vi "test-translation3d.vi"(8 "error in (no error)":errorcluster) -> (0 "error out":errorcluster, 3 "All PASSED":bool)   [LabVIEW 2019]
uses:
  <vilib>/Rock Robotics/WPI/ThirdParty/JAS_Junk/TrajLib/VI/Quaternion_New.vi
  <vilib>/Rock Robotics/WPI/ThirdParty/JAS_Junk/TrajLib/VI/Rotation3d_Create_Default.vi
  <vilib>/Rock Robotics/WPI/ThirdParty/JAS_Junk/TrajLib/VI/Vector_Norm.vi
  <vilib>/Rock Robotics/WPI/ThirdParty/JAS_Junk/TrajLib/VecBuilder_ArrayBy1Fill.vi
  <vilib>/Rock Robotics/WPI/ThirdParty/JAS_Junk/TrajLib/VI/Rotation3d_GetQuaterion.vi
  <vilib>/Rock Robotics/WPI/ThirdParty/JAS_Junk/TrajLib/VI/Quaternion_Times.vi
  <vilib>/Rock Robotics/WPI/ThirdParty/JAS_Junk/TrajLib/VI/Quaternion_Inverse.vi
  <vilib>/Rock Robotics/WPI/ThirdParty/JAS_Junk/TrajLib/VI/Quaternion_Get_All.vi
  <vilib>/Rock Robotics/WPI/ThirdParty/JAS_Junk/TrajLib/VI/Quaternion_New_Default.vi
  <vilib>/Rock Robotics/WPI/ThirdParty/JAS_Junk/TrajLib/MatBuilder_Create.vi
  <vilib>/Rock Robotics/WPI/ThirdParty/JAS_Junk/TrajLib/Trajectory_Library.lvlib
panel:
  out "Test 7 Nearest To":bool
  out "Test 6":bool
  out "Test 3c":bool
  out "Test 3b":bool
  out "Test 3a":bool
  # "Translation3d"
  # "Didn't implement divide"
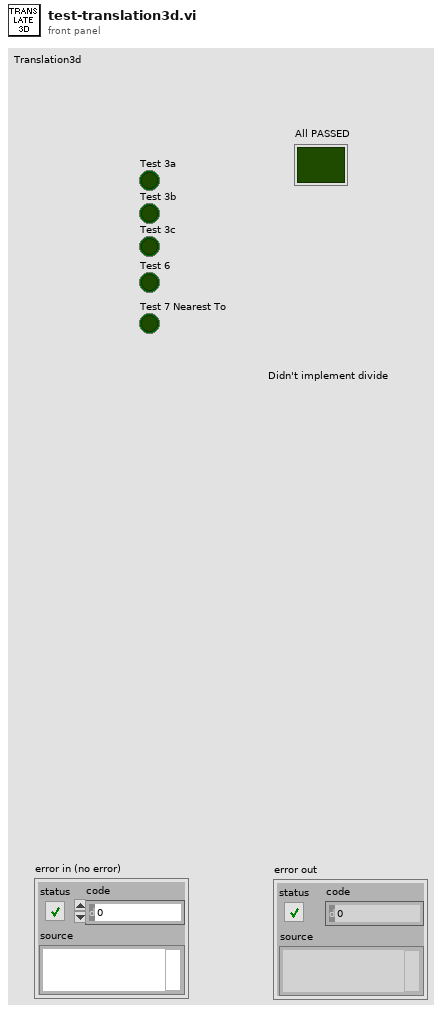
[diagram p1: front panel]
types:
  T1 = typedef "Trajectory_Library.lvlib/TRANSLATION3D.ctl" = cluster{"X":dbl, "Y":dbl, "Z":dbl}
  T2 = typedef "Trajectory_Library.lvlib/ROTATION3D.ctl" = cluster{"Q_quaternion":T3}
  T3 = typedef "Trajectory_Library.lvlib/QUATERNION.ctl" = cluster{"R":dbl, "V":dbl[]}
  T4 = typedef "Trajectory_Library.lvlib/TRANSLATION2D.ctl" = cluster{"X":dbl, "Y":dbl}
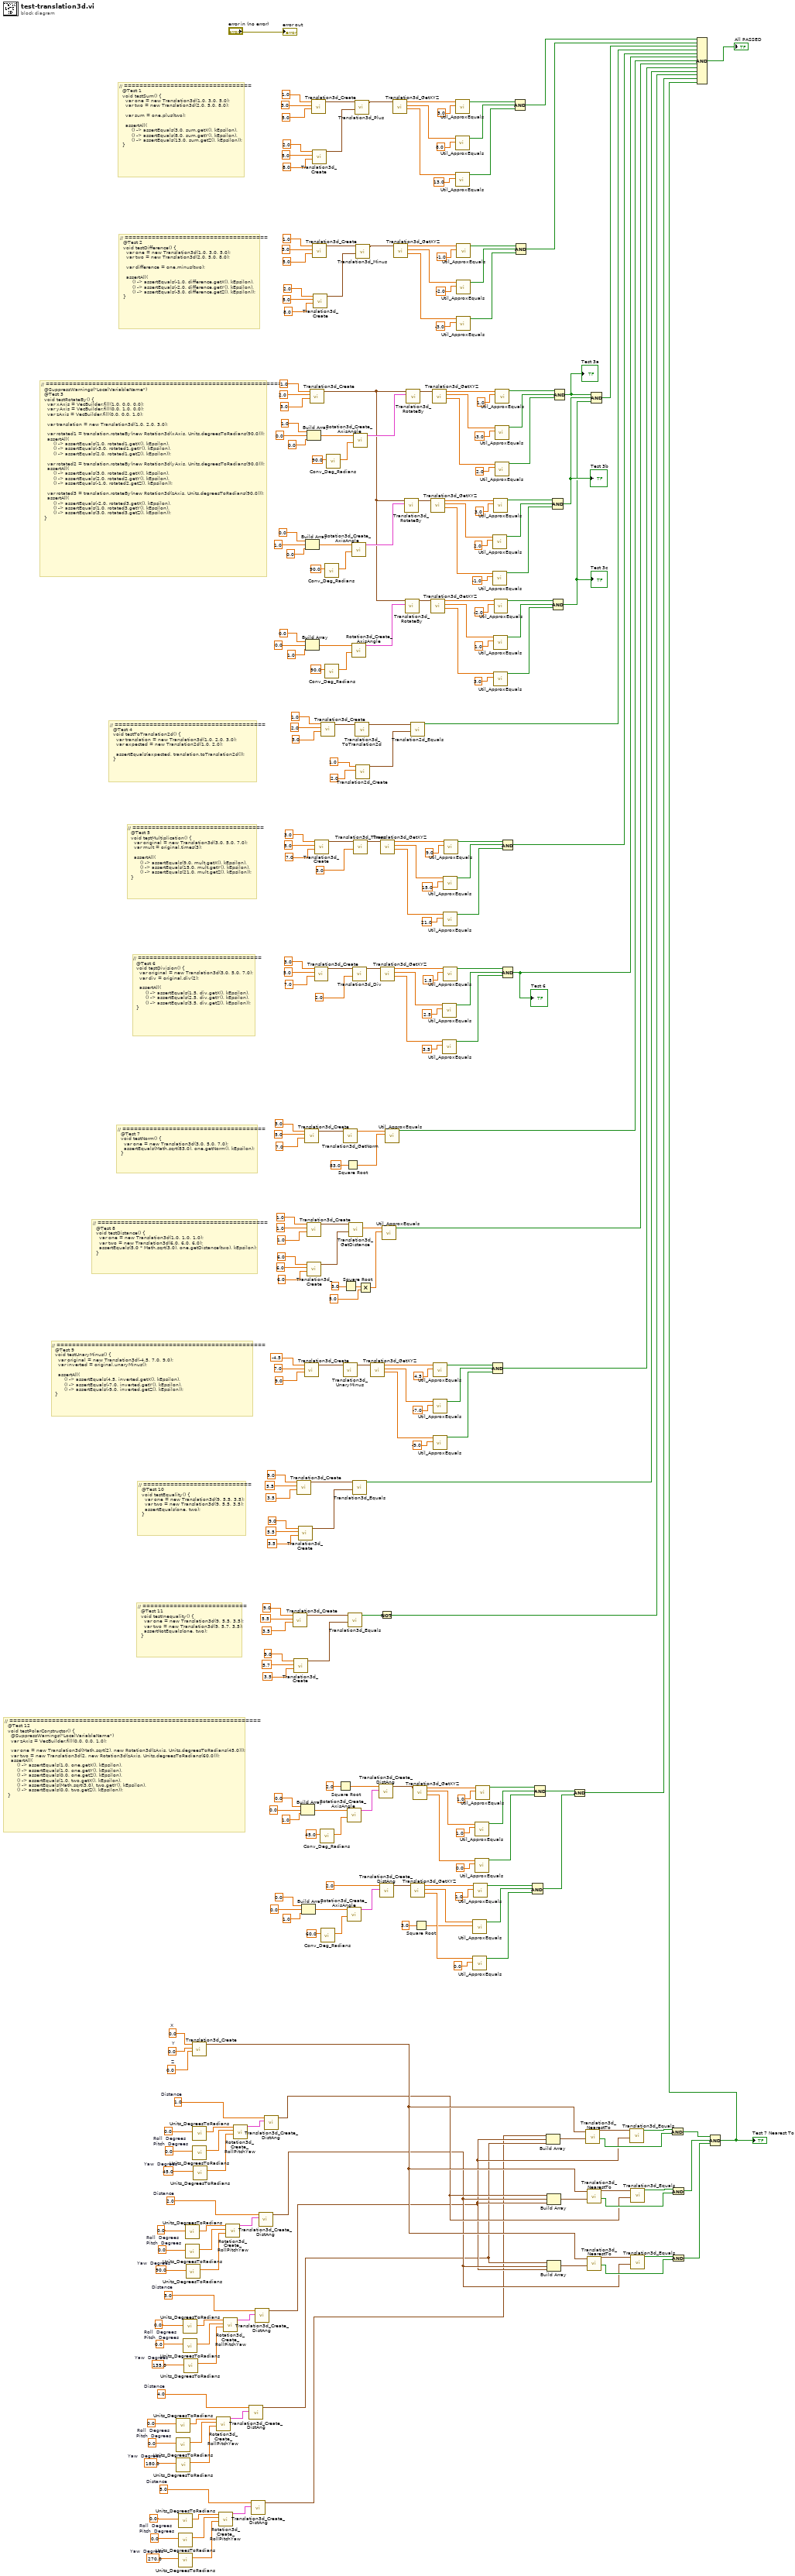
[diagram p0: block diagram]
diagram:
  w8 = 5.0  # Distance
  w10 = 0.0  # Roll  Degrees
  w11 = 0.0  # Pitch  Degrees
  w12 = 270.0  # Yaw  Degrees
  w16 = 4.0  # Distance
  w18 = 0.0  # Roll  Degrees
  w19 = 0.0  # Pitch  Degrees
  w20 = 180.0  # Yaw  Degrees
  w24 = 3.0  # Distance
  w26 = 0.0  # Roll  Degrees
  w27 = 0.0  # Pitch  Degrees
  w28 = 135.0  # Yaw  Degrees
  w32 = 2.0  # Distance
  w34 = 0.0  # Roll  Degrees
  w35 = 0.0  # Pitch  Degrees
  w36 = 90.0  # Yaw  Degrees
  w40 = 1.0  # Distance
  w42 = 0.0  # Roll  Degrees
  w43 = 0.0  # Pitch  Degrees
  w44 = 45.0  # Yaw  Degrees
  w50 = 0.0  # Z
  w49 = 0.0  # X
  w48 = 0.0  # Y
  # "// =================================================================\n  @Test 12\n  void testPolarConstructor() {\n    @SuppressWarnings(\"LocalVariableName\")\n    var zAxis = VecBuilder.fill(0.0, 0.0, 1.0);\n\n    var one = new Translation3d(Math.sqrt(2), new Rotation3d(zAxis, Units.degreesToRadians(45.0)));\n    var two = new Translation3d(2, new Rotation3d(zAxis, Units.degreesToRadians(60.0)));\n    assertAll(\n        () -> assertEquals(1.0, one.getX(), kEpsilon),\n        () -> assertEquals(1.0, one.getY(), kEpsilon),\n        () -> assertEquals(0.0, one.getZ(), kEpsilon),\n        () -> assertEquals(1.0, two.getX(), kEpsilon),\n        () -> assertEquals(Math.sqrt(3.0), two.getY(), kEpsilon),\n        () -> assertEquals(0.0, two.getZ(), kEpsilon));\n  }"
  # "// ===========================\n  @Test 11\n  void testInequality() {\n    var one = new Translation3d(9, 5.5, 3.5);\n    var two = new Translation3d(9, 5.7, 3.5);\n    assertNotEquals(one, two);\n  }"
  # "// ============================\n  @Test 10\n  void testEquality() {\n    var one = new Translation3d(9, 5.5, 3.5);\n    var two = new Translation3d(9, 5.5, 3.5);\n    assertEquals(one, two);\n  }"
  # "// ======================================================\n  @Test 9\n  void testUnaryMinus() {\n    var original = new Translation3d(-4.5, 7.0, 9.0);\n    var inverted = original.unaryMinus();\n\n    assertAll(\n        () -> assertEquals(4.5, inverted.getX(), kEpsilon),\n        () -> assertEquals(-7.0, inverted.getY(), kEpsilon),\n        () -> assertEquals(-9.0, inverted.getZ(), kEpsilon));\n  }"
  # "// ============================================\n  @Test 8\n  void testDistance() {\n    var one = new Translation3d(1.0, 1.0, 1.0);\n    var two = new Translation3d(6.0, 6.0, 6.0);\n    assertEquals(5.0 * Math.sqrt(3.0), one.getDistance(two), kEpsilon);\n  }"
  # "// =====================================\n  @Test 7\n  void testNorm() {\n    var one = new Translation3d(3.0, 5.0, 7.0);\n    assertEquals(Math.sqrt(83.0), one.getNorm(), kEpsilon);\n  }"
  # "// ================================\n  @Test 6\n  void testDivision() {\n    var original = new Translation3d(3.0, 5.0, 7.0);\n    var div = original.div(2);\n\n    assertAll(\n        () -> assertEquals(1.5, div.getX(), kEpsilon),\n        () -> assertEquals(2.5, div.getY(), kEpsilon),\n        () -> assertEquals(3.5, div.getZ(), kEpsilon));\n  }"
  # "// ==================================\n  @Test 5\n  void testMultiplication() {\n    var original = new Translation3d(3.0, 5.0, 7.0);\n    var mult = original.times(3);\n\n    assertAll(\n        () -> assertEquals(9.0, mult.getX(), kEpsilon),\n        () -> assertEquals(15.0, mult.getY(), kEpsilon),\n        () -> assertEquals(21.0, mult.getZ(), kEpsilon));\n  }"
  # "// =======================================\n  @Test 4\n  void testToTranslation2d() {\n    var translation = new Translation3d(1.0, 2.0, 3.0);\n    var expected = new Translation2d(1.0, 2.0);\n\n    assertEquals(expected, translation.toTranslation2d());\n  }"
  # "// =============================================================\n  @SuppressWarnings(\"LocalVariableName\")\n  @Test 3\n  void testRotateBy() {\n    var xAxis = VecBuilder.fill(1.0, 0.0, 0.0);\n    var yAxis = VecBuilder.fill(0.0, 1.0, 0.0);\n    var zAxis = VecBuilder.fill(0.0, 0.0, 1.0);\n\n    var translation = new Translation3d(1.0, 2.0, 3.0);\n\n    var rotated1 = translation.rotateBy(new Rotation3d(xAxis, Units.degreesToRadians(90.0)));\n    assertAll(\n        () -> assertEquals(1.0, rotated1.getX(), kEpsilon),\n        () -> assertEquals(-3.0, rotated1.getY(), kEpsilon),\n        () -> assertEquals(2.0, rotated1.getZ(), kEpsilon));\n\n    var rotated2 = translation.rotateBy(new Rotation3d(yAxis, Units.degreesToRadians(90.0)));\n    assertAll(\n        () -> assertEquals(3.0, rotated2.getX(), kEpsilon),\n        () -> assertEquals(2.0, rotated2.getY(), kEpsilon),\n        () -> assertEquals(-1.0, rotated2.getZ(), kEpsilon));\n\n    var rotated3 = translation.rotateBy(new Rotation3d(zAxis, Units.degreesToRadians(90.0)));\n    assertAll(\n        () -> assertEquals(-2.0, rotated3.getX(), kEpsilon),\n        () -> assertEquals(1.0, rotated3.getY(), kEpsilon),\n        () -> assertEquals(3.0, rotated3.getZ(), kEpsilon));\n  }"
  # "// =====================================\n  @Test 2\n  void testDifference() {\n    var one = new Translation3d(1.0, 3.0, 5.0);\n    var two = new Translation3d(2.0, 5.0, 8.0);\n\n    var difference = one.minus(two);\n\n    assertAll(\n        () -> assertEquals(-1.0, difference.getX(), kEpsilon),\n        () -> assertEquals(-2.0, difference.getY(), kEpsilon),\n        () -> assertEquals(-3.0, difference.getZ(), kEpsilon));\n  }"
  # "// =================================\n  @Test 1\n  void testSum() {\n    var one = new Translation3d(1.0, 3.0, 5.0);\n    var two = new Translation3d(2.0, 5.0, 8.0);\n\n    var sum = one.plus(two);\n\n    assertAll(\n        () -> assertEquals(3.0, sum.getX(), kEpsilon),\n        () -> assertEquals(8.0, sum.getY(), kEpsilon),\n        () -> assertEquals(13.0, sum.getZ(), kEpsilon));\n  }"
  n1 = call <vilib>:"Units_DegreesToRadians.vi"("Degrees"=w18) -> ("Radians"=w21:dbl)  [unwired: 10 in]
  n2 = call <vilib>:"Units_DegreesToRadians.vi"("Degrees"=w19) -> ("Radians"=w22:dbl)  [unwired: 10 in]
  n3 = call <vilib>:"Units_DegreesToRadians.vi"("Degrees"=w20) -> ("Radians"=w23:dbl)  [unwired: 10 in]
  n4 = call <vilib>:"Units_DegreesToRadians.vi"("Degrees"=w10) -> ("Radians"=w13:dbl)  [unwired: 10 in]
  n5 = call <vilib>:"Units_DegreesToRadians.vi"("Degrees"=w11) -> ("Radians"=w14:dbl)  [unwired: 10 in]
  n6 = call <vilib>:"Units_DegreesToRadians.vi"("Degrees"=w12) -> ("Radians"=w15:dbl)  [unwired: 10 in]
  n7 = call <vilib>:"Units_DegreesToRadians.vi"("Degrees"=w26) -> ("Radians"=w29:dbl)  [unwired: 10 in]
  n8 = call <vilib>:"Units_DegreesToRadians.vi"("Degrees"=w27) -> ("Radians"=w30:dbl)  [unwired: 10 in]
  n9 = call <vilib>:"Units_DegreesToRadians.vi"("Degrees"=w28) -> ("Radians"=w31:dbl)  [unwired: 10 in]
  n10 = call <vilib>:"Units_DegreesToRadians.vi"("Degrees"=w34) -> ("Radians"=w37:dbl)  [unwired: 10 in]
  n11 = call <vilib>:"Units_DegreesToRadians.vi"("Degrees"=w35) -> ("Radians"=w38:dbl)  [unwired: 10 in]
  n12 = call <vilib>:"Units_DegreesToRadians.vi"("Degrees"=w36) -> ("Radians"=w39:dbl)  [unwired: 10 in]
  n13 = call <vilib>:"Translation3d_Create.vi"("Z"=w50, "Y"=w48, "X"=w49) -> ("TRANSLATION3D"=w7:T1)  [unwired: 8 in]
  n14 = call <vilib>:"Units_DegreesToRadians.vi"("Degrees"=w42) -> ("Radians"=w45:dbl)  [unwired: 10 in]
  n15 = call <vilib>:"Units_DegreesToRadians.vi"("Degrees"=w43) -> ("Radians"=w46:dbl)  [unwired: 10 in]
  n16 = call <vilib>:"Units_DegreesToRadians.vi"("Degrees"=w44) -> ("Radians"=w47:dbl)  [unwired: 10 in]
  n17 = call <vilib>:"Rotation3d_Create_RollPitchYaw.vi"("Yaw"=w23, "Pitch"=w22, "Roll"=w21) -> ("Rotation3d"=w17:T2)  [unwired: 8 in]
  n18 = call <vilib>:"Rotation3d_Create_RollPitchYaw.vi"("Yaw"=w15, "Pitch"=w14, "Roll"=w13) -> ("Rotation3d"=w9:T2)  [unwired: 8 in]
  n19 = call <vilib>:"Rotation3d_Create_RollPitchYaw.vi"("Yaw"=w31, "Pitch"=w30, "Roll"=w29) -> ("Rotation3d"=w25:T2)  [unwired: 8 in]
  n20 = call <vilib>:"Rotation3d_Create_RollPitchYaw.vi"("Yaw"=w39, "Pitch"=w38, "Roll"=w37) -> ("Rotation3d"=w33:T2)  [unwired: 8 in]
  n21 = call <vilib>:"Rotation3d_Create_RollPitchYaw.vi"("Yaw"=w47, "Pitch"=w46, "Roll"=w45) -> ("Rotation3d"=w41:T2)  [unwired: 8 in]
  n22 = call <vilib>:"Translation3d_Create_DistAng.vi"("Angle_Rotation3d"=w17, "Distance"=w16) -> ("TRANSLATION3D"=w3:T1)  [unwired: 9 in]
  n23 = call <vilib>:"Translation3d_Create_DistAng.vi"("Angle_Rotation3d"=w9, "Distance"=w8) -> ("TRANSLATION3D"=w2:T1)  [unwired: 9 in]
  n24 = call <vilib>:"Translation3d_Create_DistAng.vi"("Angle_Rotation3d"=w25, "Distance"=w24) -> ("TRANSLATION3D"=w4:T1)  [unwired: 9 in]
  n25 = call <vilib>:"Translation3d_Create_DistAng.vi"("Angle_Rotation3d"=w33, "Distance"=w32) -> ("TRANSLATION3D"=w5:T1)  [unwired: 9 in]
  n26 = call <vilib>:"Translation3d_Create_DistAng.vi"("Angle_Rotation3d"=w41, "Distance"=w40) -> ("TRANSLATION3D"=w6:T1)  [unwired: 9 in]
  n27 = call <vilib>:"Translation3d_Create.vi"("Z"=3.5, "Y"=5.5, "X"=9.0) -> ("TRANSLATION3D"=w110:T1)  [unwired: 8 in]
  n28 = call <vilib>:"Translation3d_Create.vi"("Z"=3.5, "Y"=5.7, "X"=9.0) -> ("TRANSLATION3D"=w109:T1)  [unwired: 8 in]
  n29 = call <vilib>:"Translation3d_Create.vi"("Z"=3.5, "Y"=5.5, "X"=9.0) -> ("TRANSLATION3D"=w119:T1)  [unwired: 8 in]
  n30 = call <vilib>:"Translation3d_Create.vi"("Z"=3.5, "Y"=5.5, "X"=9.0) -> ("TRANSLATION3D"=w118:T1)  [unwired: 8 in]
  n31 = Build Array(0.0 ("element"), 0.0 ("element"), 1.0 ("element")) -> (w103:dbl[])
  n32 = Build Array(0.0 ("element"), 0.0 ("element"), 1.0 ("element")) -> (w94:dbl[])
  n33 = call <vilib>:"Translation3d_Create.vi"("Z"=9.0, "Y"=7.0, "X"=-4.5) -> ("TRANSLATION3D"=w137:T1)  [unwired: 8 in]
  n34 = call <vilib>:"Translation3d_Create.vi"("Z"=7.0, "Y"=5.0, "X"=3.0) -> ("TRANSLATION3D"=w159:T1)  [unwired: 8 in]
  n35 = Build Array(0.0 ("element"), 1.0 ("element"), 0.0 ("element")) -> (w239:dbl[])
  n36 = Build Array(0.0 ("element"), 0.0 ("element"), 1.0 ("element")) -> (w222:dbl[])
  n37 = call <vilib>:"Translation3d_Create.vi"("Z"=1.0, "Y"=1.0, "X"=1.0) -> ("TRANSLATION3D"=w148:T1)  [unwired: 8 in]
  n38 = Build Array(1.0 ("element"), 0.0 ("element"), 0.0 ("element")) -> (w256:dbl[])
  n39 = call <vilib>:"Translation3d_Create.vi"("Z"=6.0, "Y"=6.0, "X"=6.0) -> ("TRANSLATION3D"=w147:T1)  [unwired: 8 in]
  n40 = call <vilib>:"Translation3d_Create.vi"("Z"=3.0, "Y"=2.0, "X"=1.0) -> ("TRANSLATION3D"=w208:T1)  [unwired: 8 in]
  n41 = call <vilib>:"Translation3d_Create.vi"("Z"=5.0, "Y"=3.0, "X"=1.0) -> ("TRANSLATION3D"=w294:T1)  [unwired: 8 in]
  n42 = call <vilib>:"Translation3d_Create.vi"("Z"=8.0, "Y"=5.0, "X"=2.0) -> ("TRANSLATION3D"=w293:T1)  [unwired: 8 in]
  n43 = call <vilib>:"Translation3d_Create.vi"("Z"=5.0, "Y"=3.0, "X"=1.0) -> ("TRANSLATION3D"=w275:T1)  [unwired: 8 in]
  n44 = call <vilib>:"Translation3d_Create.vi"("Z"=8.0, "Y"=5.0, "X"=2.0) -> ("TRANSLATION3D"=w274:T1)  [unwired: 8 in]
  n45 = call <vilib>:"Translation3d_Create.vi"("Z"=7.0, "Y"=5.0, "X"=3.0) -> ("TRANSLATION3D"=w175:T1)  [unwired: 8 in]
  n46 = call <vilib>:"Translation3d_Create.vi"("Z"=7.0, "Y"=5.0, "X"=3.0) -> ("TRANSLATION3D"=w191:T1)  [unwired: 8 in]
  n47 = call <vilib>:"Conv_Deg_Radians.vi"("Degress"=45.0) -> ("Radians"=w101:dbl)  [unwired: 10 in]
  n48 = call <vilib>:"Conv_Deg_Radians.vi"("Degress"=60.0) -> ("Radians"=w92:dbl)  [unwired: 10 in]
  n49 = call <vilib>:"Translation3d_Create.vi"("Z"=3.0, "Y"=2.0, "X"=1.0) -> ("TRANSLATION3D"=w200:T1)  [unwired: 8 in]
  n50 = call <vilib>:"Conv_Deg_Radians.vi"("Degress"=90.0) -> ("Radians"=w237:dbl)  [unwired: 10 in]
  n51 = call <vilib>:"Conv_Deg_Radians.vi"("Degress"=90.0) -> ("Radians"=w220:dbl)  [unwired: 10 in]
  n52 = call <vilib>:"Conv_Deg_Radians.vi"("Degress"=90.0) -> ("Radians"=w254:dbl)  [unwired: 10 in]
  n53 = Square Root(x=2.0) -> (sqrt(x)=w98:dbl)
  n54 = call <vilib>:"Translation3d_UnaryMinus.vi"("In Translation3d"=w137) -> ("Out Translation3d"=w127:T1)  [unwired: 10 in]
  n55 = call <vilib>:"Translation3d_GetNorm.vi"("In Translation3d"=w159) -> ("Norm"=w157:dbl)  [unwired: 10 in]
  n56 = Square Root(x=3.0) -> (sqrt(x)=w144:dbl)
  n57 = Square Root(x=83.0) -> (sqrt(x)=w156:dbl)
  n58 = call <vilib>:"Rotation3d_Create_AxisAngle.vi"("Angle"=w101, "Axis Vector"=w103) -> ("Rotation3d"=w99:T2)  [unwired: 9 in]
  n59 = call <vilib>:"Rotation3d_Create_AxisAngle.vi"("Angle"=w92, "Axis Vector"=w94) -> ("Rotation3d"=w91:T2)  [unwired: 9 in]
  n60 = call <vilib>:"Translation3d_Equals.vi"("other Translation3d"=w109, "In Translation3d"=w110) -> ("Equals"=w108:bool)  [unwired: 9 in]
  n61 = call <vilib>:"Translation3d_GetDistance.vi"("other Translation3d"=w147, "In Translation3d"=w148) -> ("Distance"=w146:dbl)  [unwired: 9 in]
  n62 = call <vilib>:"Rotation3d_Create_AxisAngle.vi"("Angle"=w237, "Axis Vector"=w239) -> ("Rotation3d"=w236:T2)  [unwired: 9 in]
  n63 = call <vilib>:"Rotation3d_Create_AxisAngle.vi"("Angle"=w220, "Axis Vector"=w222) -> ("Rotation3d"=w219:T2)  [unwired: 9 in]
  n64 = call <vilib>:"Translation3d_Equals.vi"("other Translation3d"=w118, "In Translation3d"=w119) -> ("Equals"=w117:bool)  [unwired: 9 in]
  n65 = call <vilib>:"Translation3d_Div.vi"("Scalar"=2.0, "In Translation3d"=w175) -> ("Out Translation3d"=w164:T1)  [unwired: 9 in]
  n66 = call <vilib>:"Rotation3d_Create_AxisAngle.vi"("Angle"=w254, "Axis Vector"=w256) -> ("Rotation3d"=w253:T2)  [unwired: 9 in]
  n67 = call <vilib>:"Translation3d_Times.vi"("Scalar"=3.0, "In Translation3d"=w191) -> ("Out Translation3d"=w180:T1)  [unwired: 9 in]
  n68 = call <vilib>:"Translation3d_Plus.vi"("other Translation3d"=w293, "In Translation3d"=w294) -> ("Out Translation3d"=w292:T1)  [unwired: 9 in]
  n69 = call <vilib>:"Translation3d_ToTranslation2d.vi"("In Translation3d"=w200) -> ("Translation2d"=w197:T4)  [unwired: 10 in]
  n70 = call <vilib>:"Translation3d_Minus.vi"("other Translation3d"=w274, "In Translation3d"=w275) -> ("Out Translation3d"=w273:T1)  [unwired: 9 in]
  n71 = call <vilib>:"Translation2d_Create.vi"("Y"=2.0, "X"=1.0) -> ("TRANSLATION"=w196:T4)  [unwired: 9 in]
  n72 = Multiply(x=w144, y=5.0) -> (x*y=w142:dbl)
  n73 = call <vilib>:"Translation3d_GetXYZ.vi"("In Translation3d"=w127) -> ("Z"=w134:dbl, "Y"=w135:dbl, "X"=w136:dbl)  [unwired: 8 in]
  n74 = call <vilib>:"Translation3d_Create_DistAng.vi"("Angle_Rotation3d"=w99, "Distance"=w98) -> ("TRANSLATION3D"=w72:T1)  [unwired: 9 in]
  n75 = call <vilib>:"Translation3d_Create_DistAng.vi"("Angle_Rotation3d"=w91, "Distance"=2.0 ("x")) -> ("TRANSLATION3D"=w73:T1)  [unwired: 9 in]
  n76 = Not(x=w108) -> (.not. x?=w107:bool)
  n77 = call <vilib>:"Translation3d_GetXYZ.vi"("In Translation3d"=w164) -> ("Z"=w171:dbl, "Y"=w172:dbl, "X"=w173:dbl)  [unwired: 8 in]
  n78 = call <vilib>:"Translation3d_GetXYZ.vi"("In Translation3d"=w180) -> ("Z"=w187:dbl, "Y"=w188:dbl, "X"=w189:dbl)  [unwired: 8 in]
  n79 = call <vilib>:"Util_ApproxEquals.vi"("Value 2"=w142, "Value 1"=w146) -> ("ApproxEquals"=w141:bool)  [unwired: 9 in]
  n80 = call <vilib>:"Util_ApproxEquals.vi"("Value 2"=w156, "Value 1"=w157) -> ("ApproxEquals"=w155:bool)  [unwired: 9 in]
  n81 = call <vilib>:"Translation3d_GetXYZ.vi"("In Translation3d"=w292) -> ("Z"=w289:dbl, "Y"=w290:dbl, "X"=w291:dbl)  [unwired: 8 in]
  n82 = call <vilib>:"Translation3d_GetXYZ.vi"("In Translation3d"=w273) -> ("Z"=w270:dbl, "Y"=w271:dbl, "X"=w272:dbl)  [unwired: 8 in]
  n83 = call <vilib>:"Translation3d_RotateBy.vi"("other Rot3d"=w236, "in Translation3D"=w208) -> ("out Translation3d"=w226:T1)  [unwired: 9 in]
  n84 = call <vilib>:"Translation3d_RotateBy.vi"("other Rot3d"=w219, "in Translation3D"=w208) -> ("out Translation3d"=w209:T1)  [unwired: 9 in]
  n85 = call <vilib>:"Translation3d_RotateBy.vi"("other Rot3d"=w253, "in Translation3D"=w208) -> ("out Translation3d"=w243:T1)  [unwired: 9 in]
  n86 = call <vilib>:"Translation3d_GetXYZ.vi"("In Translation3d"=w73) -> ("Z"=w79:dbl, "Y"=w80:dbl, "X"=w81:dbl)  [unwired: 8 in]
  n87 = call <vilib>:"Translation2d_Equals.vi"("other Translation"=w196, "In Translation"=w197) -> ("Equals"=w195:bool)  [unwired: 9 in]
  n88 = call <vilib>:"Translation3d_GetXYZ.vi"("In Translation3d"=w72) -> ("Z"=w88:dbl, "Y"=w89:dbl, "X"=w90:dbl)  [unwired: 8 in]
  n89 = Square Root(x=3.0) -> (sqrt(x)=w69:dbl)
  n90 = call <vilib>:"Translation3d_GetXYZ.vi"("In Translation3d"=w226) -> ("Z"=w233:dbl, "Y"=w234:dbl, "X"=w235:dbl)  [unwired: 8 in]
  n91 = call <vilib>:"Translation3d_GetXYZ.vi"("In Translation3d"=w209) -> ("Z"=w216:dbl, "Y"=w217:dbl, "X"=w218:dbl)  [unwired: 8 in]
  n92 = call <vilib>:"Translation3d_GetXYZ.vi"("In Translation3d"=w243) -> ("Z"=w250:dbl, "Y"=w251:dbl, "X"=w252:dbl)  [unwired: 8 in]
  n93 = call <vilib>:"Util_ApproxEquals.vi"("Value 2"=-7.0, "Value 1"=w135) -> ("ApproxEquals"=w129:bool)  [unwired: 9 in]
  n94 = call <vilib>:"Util_ApproxEquals.vi"("Value 2"=-9.0, "Value 1"=w134) -> ("ApproxEquals"=w128:bool)  [unwired: 9 in]
  n95 = call <vilib>:"Util_ApproxEquals.vi"("Value 2"=4.5, "Value 1"=w136) -> ("ApproxEquals"=w130:bool)  [unwired: 9 in]
  n96 = call <vilib>:"Util_ApproxEquals.vi"("Value 2"=2.5, "Value 1"=w172) -> ("ApproxEquals"=w166:bool)  [unwired: 9 in]
  n97 = call <vilib>:"Util_ApproxEquals.vi"("Value 2"=3.5, "Value 1"=w171) -> ("ApproxEquals"=w165:bool)  [unwired: 9 in]
  n98 = call <vilib>:"Util_ApproxEquals.vi"("Value 2"=15.0, "Value 1"=w188) -> ("ApproxEquals"=w182:bool)  [unwired: 9 in]
  n99 = call <vilib>:"Util_ApproxEquals.vi"("Value 2"=21.0, "Value 1"=w187) -> ("ApproxEquals"=w181:bool)  [unwired: 9 in]
  n100 = call <vilib>:"Util_ApproxEquals.vi"("Value 2"=1.5, "Value 1"=w173) -> ("ApproxEquals"=w167:bool)  [unwired: 9 in]
  n101 = call <vilib>:"Util_ApproxEquals.vi"("Value 2"=9.0, "Value 1"=w189) -> ("ApproxEquals"=w183:bool)  [unwired: 9 in]
  n102 = call <vilib>:"Util_ApproxEquals.vi"("Value 2"=8.0, "Value 1"=w290) -> ("ApproxEquals"=w284:bool)  [unwired: 9 in]
  n103 = call <vilib>:"Util_ApproxEquals.vi"("Value 2"=13.0, "Value 1"=w289) -> ("ApproxEquals"=w283:bool)  [unwired: 9 in]
  n104 = call <vilib>:"Util_ApproxEquals.vi"("Value 2"=3.0, "Value 1"=w291) -> ("ApproxEquals"=w285:bool)  [unwired: 9 in]
  n105 = call <vilib>:"Util_ApproxEquals.vi"("Value 2"=-2.0, "Value 1"=w271) -> ("ApproxEquals"=w265:bool)  [unwired: 9 in]
  n106 = call <vilib>:"Util_ApproxEquals.vi"("Value 2"=-3.0, "Value 1"=w270) -> ("ApproxEquals"=w264:bool)  [unwired: 9 in]
  n107 = call <vilib>:"Util_ApproxEquals.vi"("Value 2"=-1.0, "Value 1"=w272) -> ("ApproxEquals"=w266:bool)  [unwired: 9 in]
  n108 = call <vilib>:"Util_ApproxEquals.vi"("Value 2"=w69, "Value 1"=w80) -> ("ApproxEquals"=w75:bool)  [unwired: 9 in]
  n109 = call <vilib>:"Util_ApproxEquals.vi"("Value 2"=0.0, "Value 1"=w79) -> ("ApproxEquals"=w74:bool)  [unwired: 9 in]
  n110 = call <vilib>:"Util_ApproxEquals.vi"("Value 2"=1.0, "Value 1"=w81) -> ("ApproxEquals"=w76:bool)  [unwired: 9 in]
  n111 = call <vilib>:"Util_ApproxEquals.vi"("Value 2"=1.0, "Value 1"=w89) -> ("ApproxEquals"=w83:bool)  [unwired: 9 in]
  n112 = call <vilib>:"Util_ApproxEquals.vi"("Value 2"=0.0, "Value 1"=w88) -> ("ApproxEquals"=w82:bool)  [unwired: 9 in]
  n113 = call <vilib>:"Util_ApproxEquals.vi"("Value 2"=1.0, "Value 1"=w90) -> ("ApproxEquals"=w84:bool)  [unwired: 9 in]
  n114 = Compound Arithmetic op=AND(w130, w129, w128) -> (w126:bool)
  n115 = call <vilib>:"Util_ApproxEquals.vi"("Value 2"=2.0, "Value 1"=w234) -> ("ApproxEquals"=w228:bool)  [unwired: 9 in]
  n116 = call <vilib>:"Util_ApproxEquals.vi"("Value 2"=-1.0, "Value 1"=w233) -> ("ApproxEquals"=w227:bool)  [unwired: 9 in]
  n117 = call <vilib>:"Util_ApproxEquals.vi"("Value 2"=3.0, "Value 1"=w235) -> ("ApproxEquals"=w229:bool)  [unwired: 9 in]
  n118 = call <vilib>:"Util_ApproxEquals.vi"("Value 2"=1.0, "Value 1"=w217) -> ("ApproxEquals"=w211:bool)  [unwired: 9 in]
  n119 = call <vilib>:"Util_ApproxEquals.vi"("Value 2"=3.0, "Value 1"=w216) -> ("ApproxEquals"=w210:bool)  [unwired: 9 in]
  n120 = call <vilib>:"Util_ApproxEquals.vi"("Value 2"=-2.0, "Value 1"=w218) -> ("ApproxEquals"=w212:bool)  [unwired: 9 in]
  n121 = call <vilib>:"Util_ApproxEquals.vi"("Value 2"=-3.0, "Value 1"=w251) -> ("ApproxEquals"=w245:bool)  [unwired: 9 in]
  n122 = call <vilib>:"Util_ApproxEquals.vi"("Value 2"=2.0, "Value 1"=w250) -> ("ApproxEquals"=w244:bool)  [unwired: 9 in]
  n123 = call <vilib>:"Util_ApproxEquals.vi"("Value 2"=1.0, "Value 1"=w252) -> ("ApproxEquals"=w246:bool)  [unwired: 9 in]
  n124 = Compound Arithmetic op=AND(w167, w166, w165) -> (w163:bool)
  "Test 6" <- w163
  n125 = Compound Arithmetic op=AND(w183, w182, w181) -> (w179:bool)
  n126 = Compound Arithmetic op=AND(w285, w284, w283) -> (w282:bool)
  n127 = Compound Arithmetic op=AND(w266, w265, w264) -> (w263:bool)
  n128 = Compound Arithmetic op=AND(w76, w75, w74) -> (w67:bool)
  n129 = Compound Arithmetic op=AND(w84, w83, w82) -> (w68:bool)
  n130 = Build Array(w2, w4, w3) -> (w65:T1[])
  n131 = Build Array(w6, w5, w4) -> (w60:T1[])
  n132 = Build Array(w3, w5, w4) -> (w56:T1[])
  n133 = Compound Arithmetic op=AND(w229, w228, w227) -> (w205:bool)
  "Test 3b" <- w205
  n134 = Compound Arithmetic op=AND(w212, w211, w210) -> (w204:bool)
  "Test 3c" <- w204
  n135 = Compound Arithmetic op=AND(w246, w245, w244) -> (w207:bool)
  "Test 3a" <- w207
  n136 = Compound Arithmetic op=AND(w68, w67) -> (w66:bool)
  n137 = call <vilib>:"Translation3d_NearestTo.vi"("Other Translation3d"=w65, "In Translation3d"=w7) -> ("Found"=w63:bool, "Nearest Translation3d"=w64:T1)  [unwired: 8 in]
  n138 = call <vilib>:"Translation3d_NearestTo.vi"("Other Translation3d"=w60, "In Translation3d"=w7) -> ("Found"=w58:bool, "Nearest Translation3d"=w59:T1)  [unwired: 8 in]
  n139 = call <vilib>:"Translation3d_NearestTo.vi"("Other Translation3d"=w56, "In Translation3d"=w7) -> ("Found"=w54:bool, "Nearest Translation3d"=w55:T1)  [unwired: 8 in]
  n140 = Compound Arithmetic op=AND(w207, w205, w204) -> (w206:bool)
  n141 = call <vilib>:"Translation3d_Equals.vi"("other Translation3d"=w4, "In Translation3d"=w64) -> ("Equals"=w62:bool)  [unwired: 9 in]
  n142 = call <vilib>:"Translation3d_Equals.vi"("other Translation3d"=w6, "In Translation3d"=w59) -> ("Equals"=w57:bool)  [unwired: 9 in]
  n143 = call <vilib>:"Translation3d_Equals.vi"("other Translation3d"=w5, "In Translation3d"=w55) -> ("Equals"=w53:bool)  [unwired: 9 in]
  n144 = And(x=w62, y=w63) -> (x .and. y?=w61:bool)
  n145 = And(x=w57, y=w58) -> (x .and. y?=w52:bool)
  n146 = And(x=w53, y=w54) -> (x .and. y?=w51:bool)
  n147 = Compound Arithmetic op=AND(w61, w52, w51) -> (w1:bool)
  "Test 7 Nearest To" <- w1
  n148 = Compound Arithmetic op=AND(w282, w263, w206, w195, w179, w163, w155, w141, w126, w117, w107, w66, w1) -> (→"All PASSED":bool)
  "error out" <- "error in (no error)"
